vi "Plot.vi"(8 "error in (no error)":errorcluster, 11 "IV in":refnum<class "IV.lvclass">) -> (0 "error out":errorcluster, 1 "IV plot":cluster{dbl[], dbl[]}[](array[cluster]), 2 "dVdI plot":cluster{dbl[], dbl[]}[](array[cluster]), 3 "IV out":refnum<class "IV.lvclass">)   [LabVIEW 2021, in "IV.lvclass"]
uses:
  IV.lvclass
  Libraries/Instruments/Results/Acquired Result/Acquired Result.lvclass
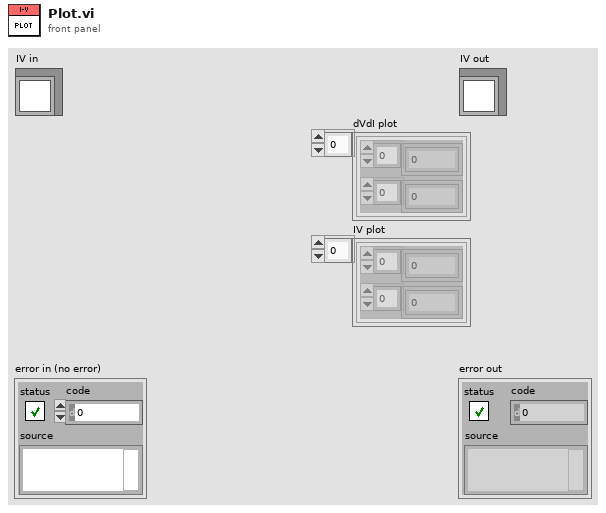
[diagram p1: front panel]
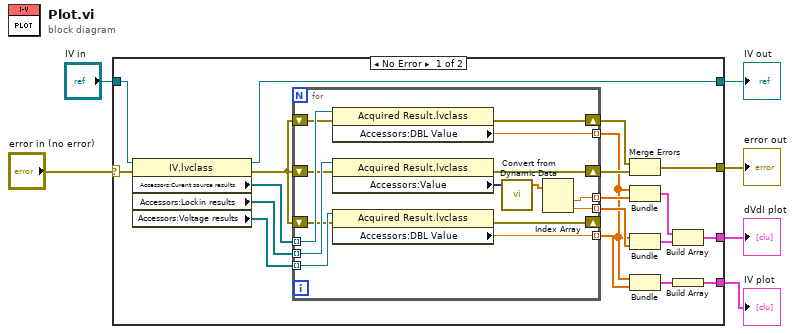
[diagram p0: block diagram]
diagram:
  n1 = case shown="No Error" "error in (no error)" {
    selector: "error in (no error)" -> [w25 w42]
    tunnel: [w15 w42] -> w5
    tunnel: [w23 w41] -> w3
    tunnel: "IV in" -> [w24 w41]
    tunnel: [w16 _] -> w2
    tunnel: [w7 _] -> w1
    frame No Error {
      n2 = property class="IV.lvclass"(reference=w24, error in=w25) -> (reference out=w23:refnum<class "IV.lvclass">, error out=w11:errorcluster, "Accessors:Curent source results"=w22:refnum<class "Acquired Result.lvclass">[], "Accessors:Lockin results"=w21:refnum<class "Acquired Result.lvclass">[], "Accessors:Voltage results"=w12:refnum<class "Acquired Result.lvclass">[])
      n3 = for {
        tunnel: w22 -> [w40] mode=indexing
        tunnel: w21 -> [w39] mode=indexing
        shift-right: [w34] -> w14
        shift-left: w11 -> [w36]
        shift-right: [w33] -> w13
        shift-left: w11 -> [w35]
        tunnel: [w32] -> w10 mode=indexing
        tunnel: [w31] -> w20 mode=indexing
        tunnel: [w30] -> w19 mode=indexing
        tunnel: w12 -> [w29] mode=indexing
        shift-right: [w27] -> _
        shift-left: w11 -> [w28]
        tunnel: [w26] -> w9 mode=indexing
        n4 = property class="Acquired Result.lvclass"(reference=w40, error in=w36) -> (error out=w34:errorcluster, "Accessors:DBL Value"=w32:dbl)  [unwired: 1 out]
        n5 = property class="Acquired Result.lvclass"(reference=w39, error in=w35) -> (error out=w33:errorcluster, "Accessors:Value"=w37:dynamicdata)  [unwired: 1 out]
        n6 = property class="Acquired Result.lvclass"(reference=w29, error in=w28) -> (error out=w27:errorcluster, "Accessors:DBL Value"=w26:dbl)  [unwired: 1 out]
        n7 = call "Convert from Dynamic Data"("Dynamic Data Type"=w37) -> ("Array"=w38:dbl[])  [unwired: 3 in]
        n8 = Index Array(array=w38) -> (element #1=w31:dbl, element #2=w30:dbl)  [unwired: 2 in]
      }
      n9 = Merge Errors(w14, w13) -> (w15:errorcluster)
      n10 = Bundle(w10, w20) -> (w18:cluster{dbl[], dbl[]})  [unwired: 1 in]
      n11 = Bundle(w10, w19) -> (w17:cluster{dbl[], dbl[]})  [unwired: 1 in]
      n12 = Bundle(w10, w9) -> (w8:cluster{dbl[], dbl[]})  [unwired: 1 in]
      n13 = Build Array(w18, w17) -> (w16:cluster{dbl[], dbl[]}[])
      n14 = Build Array(w8) -> (w7:cluster{dbl[], dbl[]}[])
    }
    frame Error {
    }
  }
  "error out" <- w5
  "IV out" <- w3
  "dVdI plot" <- w2
  "IV plot" <- w1
